vi "Value_check.vi"(0 "VISA引用句柄输入":refnum<visa-resource-name>, 1 "Status Code":string, 5 "错误输入（无错误）":errorcluster) -> (3 "电压设置回读":string, 4 "电流值回读":string, 6 "过温":string="CC", 7 "蜂鸣器":string="CC", 10 "测量模式":string="CC", 11 "过压":string="CC", 12 "CC/CV":string="CC", 13 "键盘锁":string="CC", 14 "电流设置回读":string, 15 "On/Off":string="CC", 16 "过压设置值回读":string, 17 "电压值回读":string, 18 "VISA资源名称输出":refnum<visa-resource-name>, 19 "错误输出":errorcluster)   [LabVIEW 2014]
panel:
  out "读取缓冲区":string
  out "连接的字符串":string
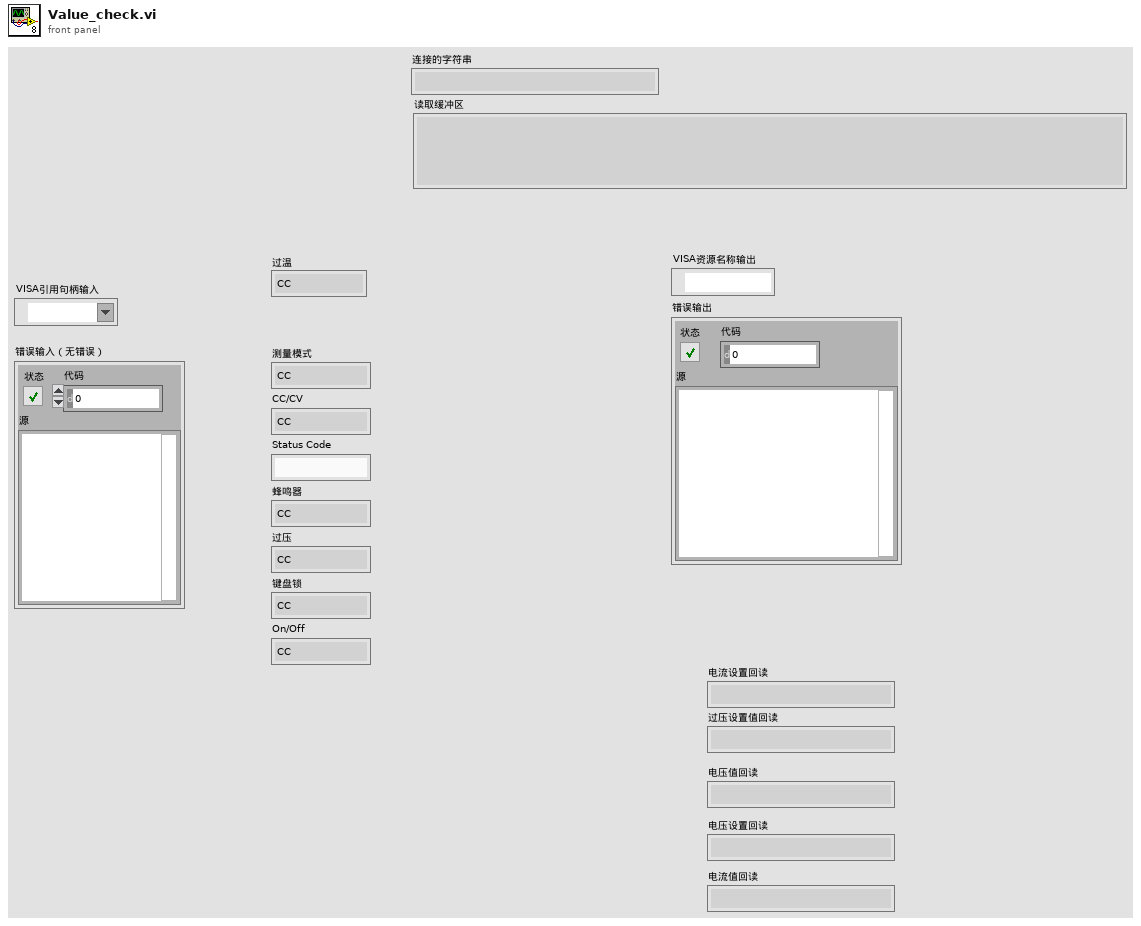
[diagram p1: front panel]
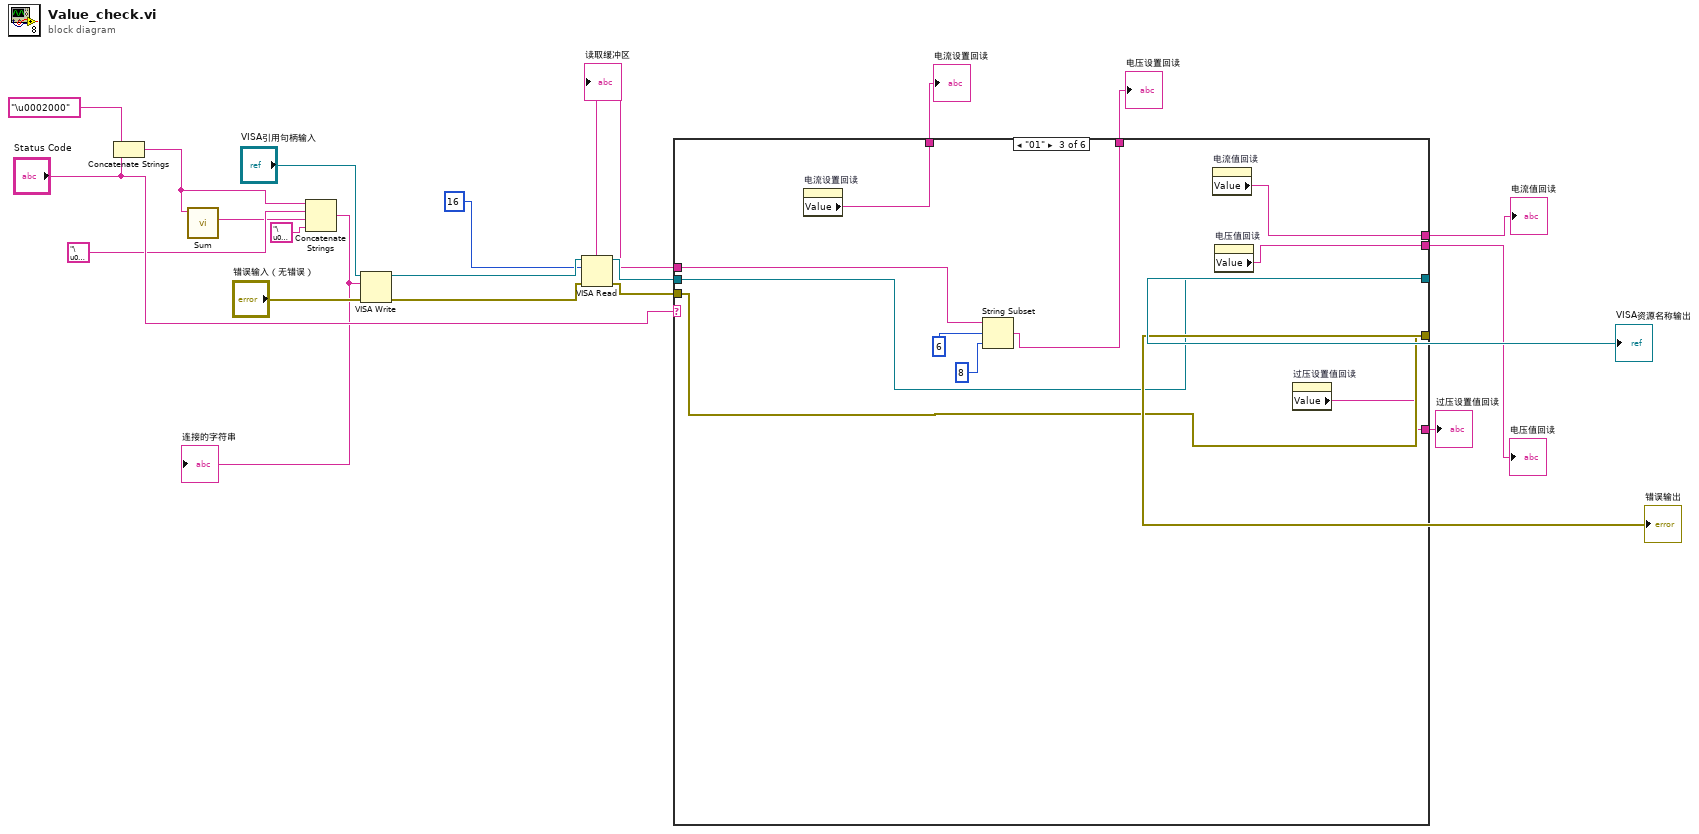
[diagram p0: block diagram]
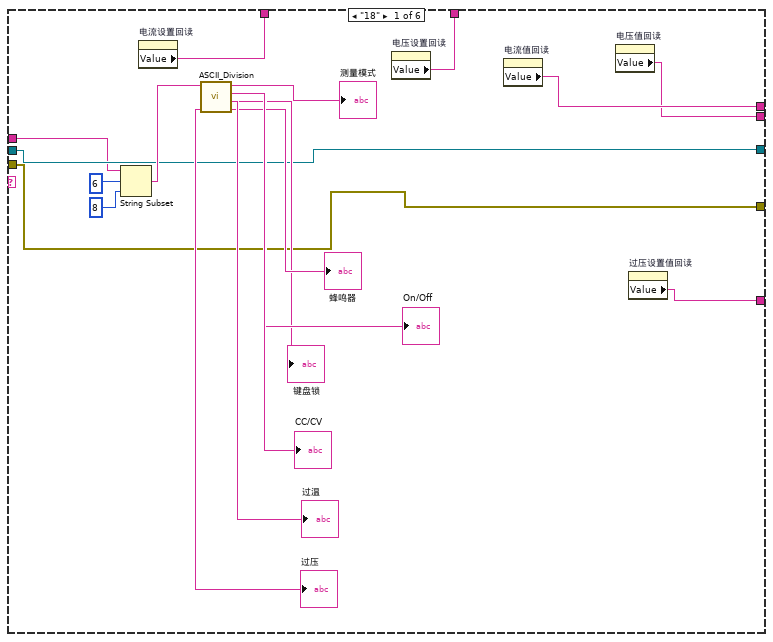
[diagram p2: hidden frame]
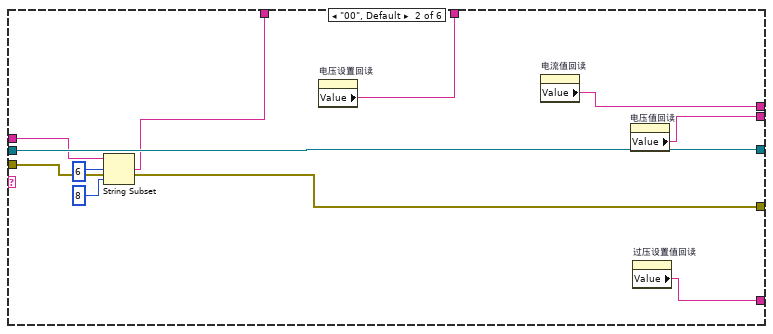
[diagram p3: hidden frame]
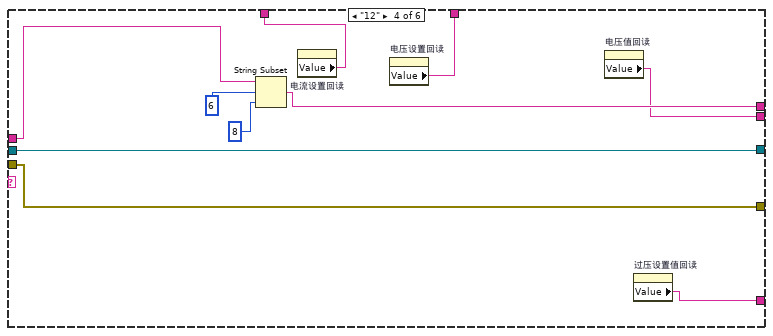
[diagram p4: hidden frame]
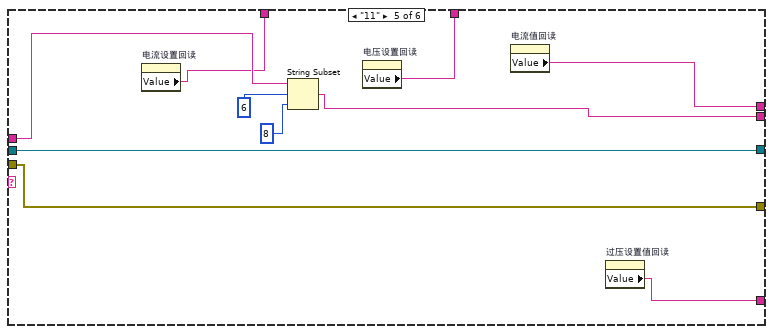
[diagram p5: hidden frame]
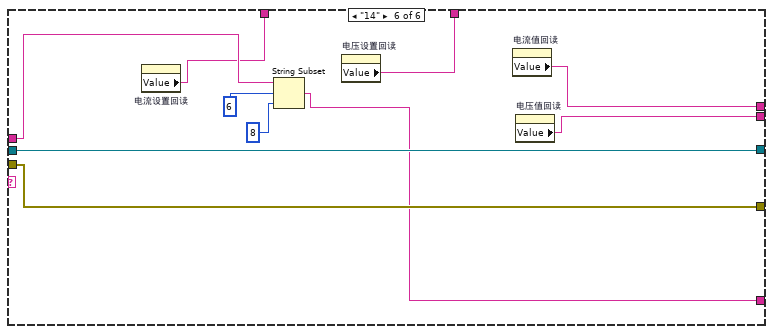
[diagram p6: hidden frame]
diagram:
  n1 = Concatenate Strings("\u0002000", "Status Code") -> (w2:string)
  n2 = call "Sum.vi"("连接的字符串"=w2) -> ("string"=w3:string)  [unwired: 8 in, 2 out]
  n3 = Concatenate Strings(w2, "\u0004", w3, "\u0003") -> (w5:string)
  "连接的字符串" <- w5
  n4 = VISA Write(VISA resource name="VISA引用句柄输入", write buffer=w5, error in (no error)="错误输入（无错误）") -> (VISA resource name out=w10:refnum<visa-resource-name>, error out=w11:errorcluster)  [unwired: 1 out]
  n5 = VISA Read(VISA resource name=w10, byte count=16, error in (no error)=w11) -> (VISA resource name out=w19:refnum<visa-resource-name>, read buffer=w17:string, error out=w18:errorcluster)  [unwired: 1 out]
  "读取缓冲区" <- w17
  n6 = case shown="\"01\"" "Status Code" {
    tunnel: w19 -> [w30 w48 w58 w70 w80 w90]
    tunnel: [w30 w48 w58 w70 w80 w90] -> w22
    tunnel: [w29 w47 w57 w69 w79 w89] -> w21
    tunnel: w18 -> [w29 w47 w57 w69 w79 w89]
    tunnel: w17 -> [w28 w46 w56 w66 w76 w86]
    tunnel: [w27 w45 w55 w65 w75 w85] -> w16
    tunnel: [w26 w44 w54 w64 w73 w83] -> w15
    tunnel: [w25 w43 w53 w63 w72 w82] -> w14
    tunnel: [w24 w42 w52 w62 w74 w81] -> w13
    tunnel: [w23 w41 w51 w61 w71 w84] -> w12
    frame "18" {
      n7 = String Subset(string=w28, offset (0)=6, length (rest)=8) -> (substring=w38:string)
      n8 = property on="电流设置回读" class="Str"() -> ("Value"=w26:string)  [unwired: 2 in, 2 out]
      n9 = call "ASCII_Division.vi"("字符串"=w38) -> ("蜂鸣器"=→"蜂鸣器":string, "键盘锁"=→"键盘锁":string, "On/Off"=→"On/Off":string, "测量模式"=→"测量模式":string, "过压"=→"过压":string, "过温"=→"过温":string, "CC/CV"=→"CC/CV":string)  [unwired: 4 in]
      n10 = property on="电压设置回读" class="Str"() -> ("Value"=w25:string)  [unwired: 2 in, 2 out]
      n11 = property on="电流值回读" class="Str"() -> ("Value"=w27:string)  [unwired: 2 in, 2 out]
      n12 = property on="电压值回读" class="Str"() -> ("Value"=w24:string)  [unwired: 2 in, 2 out]
      n13 = property on="过压设置值回读" class="Str"() -> ("Value"=w23:string)  [unwired: 2 in, 2 out]
    }
    frame "00", Default {
      n14 = String Subset(string=w46, offset (0)=6, length (rest)=8) -> (substring=w44:string)
      n15 = property on="电压设置回读" class="Str"() -> ("Value"=w43:string)  [unwired: 2 in, 2 out]
      n16 = property on="电流值回读" class="Str"() -> ("Value"=w45:string)  [unwired: 2 in, 2 out]
      n17 = property on="电压值回读" class="Str"() -> ("Value"=w42:string)  [unwired: 2 in, 2 out]
      n18 = property on="过压设置值回读" class="Str"() -> ("Value"=w41:string)  [unwired: 2 in, 2 out]
    }
    frame "01" {
      n19 = property on="电流设置回读" class="Str"() -> ("Value"=w54:string)  [unwired: 2 in, 2 out]
      n20 = String Subset(string=w56, offset (0)=6, length (rest)=8) -> (substring=w53:string)
      n21 = property on="电流值回读" class="Str"() -> ("Value"=w55:string)  [unwired: 2 in, 2 out]
      n22 = property on="电压值回读" class="Str"() -> ("Value"=w52:string)  [unwired: 2 in, 2 out]
      n23 = property on="过压设置值回读" class="Str"() -> ("Value"=w51:string)  [unwired: 2 in, 2 out]
    }
    frame "12" {
      n24 = String Subset(string=w66, offset (0)=6, length (rest)=8) -> (substring=w65:string)
      n25 = property on="电流设置回读" class="Str"() -> ("Value"=w64:string)  [unwired: 2 in, 2 out]
      n26 = property on="电压设置回读" class="Str"() -> ("Value"=w63:string)  [unwired: 2 in, 2 out]
      n27 = property on="电压值回读" class="Str"() -> ("Value"=w62:string)  [unwired: 2 in, 2 out]
      n28 = property on="过压设置值回读" class="Str"() -> ("Value"=w61:string)  [unwired: 2 in, 2 out]
    }
    frame "11" {
      n29 = property on="电流设置回读" class="Str"() -> ("Value"=w73:string)  [unwired: 2 in, 2 out]
      n30 = String Subset(string=w76, offset (0)=6, length (rest)=8) -> (substring=w74:string)
      n31 = property on="电压设置回读" class="Str"() -> ("Value"=w72:string)  [unwired: 2 in, 2 out]
      n32 = property on="电流值回读" class="Str"() -> ("Value"=w75:string)  [unwired: 2 in, 2 out]
      n33 = property on="过压设置值回读" class="Str"() -> ("Value"=w71:string)  [unwired: 2 in, 2 out]
    }
    frame "14" {
      n34 = property on="电流设置回读" class="Str"() -> ("Value"=w83:string)  [unwired: 2 in, 2 out]
      n35 = String Subset(string=w86, offset (0)=6, length (rest)=8) -> (substring=w84:string)
      n36 = property on="电压设置回读" class="Str"() -> ("Value"=w82:string)  [unwired: 2 in, 2 out]
      n37 = property on="电流值回读" class="Str"() -> ("Value"=w85:string)  [unwired: 2 in, 2 out]
      n38 = property on="电压值回读" class="Str"() -> ("Value"=w81:string)  [unwired: 2 in, 2 out]
    }
  }
  "VISA资源名称输出" <- w22
  "错误输出" <- w21
  "电流值回读" <- w16
  "电流设置回读" <- w15
  "电压设置回读" <- w14
  "电压值回读" <- w13
  "过压设置值回读" <- w12
